vi "Assert Key is Correct.vi"(5 "Assert Only? (F)":bool, 6 "error code (1)":i32=1, 7 "Label":string="Key is correct", 8 "Error In":errorcluster, 10 "Expected":string, 11 "Token":refnum<class "Abstract.lvclass">) -> (0 "Error Out":errorcluster)   [LabVIEW 2018, in "Tests.lvlib"]
uses:
  Tests.lvlib
  src/Toolkit/Low-Level/Tokens/Abstract/Abstract.lvclass
  src/Toolkit/Low-Level/Tokens/Keyable/API/Keyable.lvclass
  src/Toolkit/Low-Level/Tokens/Keyable/API/Keyable.lvclass/Keyable.ctl
  <vilib>/addons/_JKI Toolkits/Caraya/classes/Assert/Assert.lvclass
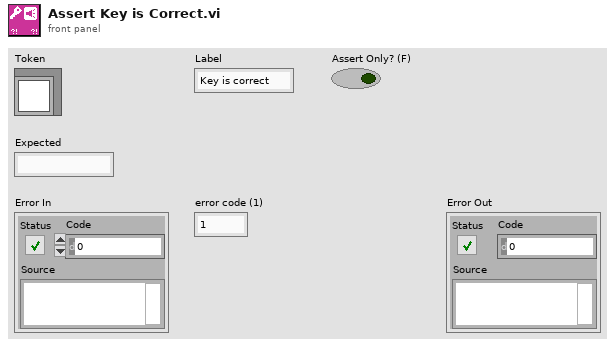
[diagram p1: front panel]
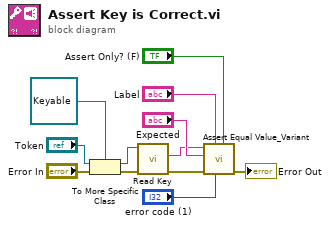
[diagram p0: block diagram]
diagram:
  n1 = To More Specific Class(target class=refnum<class "Keyable.lvclass"> refnum ("Mustache.lvlib:Tokens.lvlib:Variable.lvclass"), reference="Token", error in="Error In") -> (specific class reference=w3:refnum<class "Keyable.lvclass">, error out=w6:errorcluster)
  n2 = call "Read Key.vi"("Error In"=w6, "Keyable In"=w3) -> ("Error Out"=w7:errorcluster, "Key"=w8:string)  [unwired: 7 in, 1 out]
  n3 = call <vilib>:"Assert Equal Value_Variant.vi"("Assert Only? (F)"="Assert Only? (F)", "error code (1)"="error code (1)", "Label"="Label", "error in (no error)"=w7, "Y"="Expected", "X"=w8) -> ("error out"=→"Error Out":errorcluster)  [unwired: 5 in]
